vi "Add Small Noise.vi"(11 "channel 1":T2) -> (3 "channel 2":T1)   [LabVIEW 2019]
doc: "Given a value coming in on a channel, disturb that value by a small amount of noise."
uses:
  <extravilib>/ChannelInstances/Stream-i32/)Channel.ctl
  <extravilib>/ChannelInstances/Stream-dbl/)Channel.ctl
  <extravilib>/ChannelInstances/Stream-i32/Read With Abort.vi
  <extravilib>/ChannelInstances/Stream-dbl/Write With Abort.vi
  <extravilib>/ChannelInstances/Stream-i32/EndpointRead.vi
  <extravilib>/ChannelInstances/Stream-dbl/Endpoint.vi
  <extravilib>/ChannelInstances/Stream-i32/)Channel.vi
  <resource>/ChannelSupport/_ChannelSupport/WaitIfNeeded.vi
  <extravilib>/ChannelInstances/Stream-dbl/)Channel.vi
  <extravilib>/ChannelInstances/Stream-i32.lvlib
  <extravilib>/ChannelInstances/Stream-dbl.lvlib
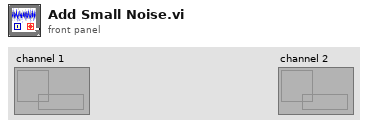
[diagram p1: front panel]
types:
  T1 = typedef "Stream-dbl.lvlib/)Channel.ctl" = refnum<queue>
  T2 = typedef "Stream-i32.lvlib/)Channel.ctl" = refnum<queue>
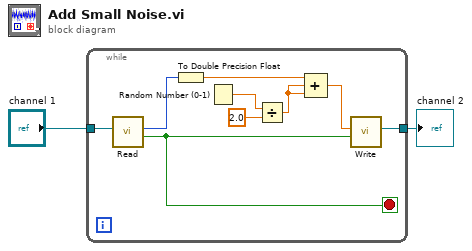
[diagram p0: block diagram]
diagram:
  n1 = while {
    tunnel: [w7] -> w1
    tunnel: "channel 1" -> [w10]
    stop <- w8 stop-if-true
    n2 = call <extravilib>:"Read.vi"("channel"=w10) -> ("last element?"=w8:bool, "element"=w9:i32)  [unwired: 6 in, 3 out]
    n3 = To Double Precision Float(number=w9) -> (double precision float=w3:dbl)
    n4 = Random Number (0-1)() -> (number: 0 to 1=w5:dbl)
    n5 = Divide(x=w5, y=2.0) -> (x/y=w4:dbl)
    n6 = Compound Arithmetic op=ADD(w3, w4, w4) -> (w11:dbl)
    n7 = call <extravilib>:"Write.vi"("last element? (F)"=w8, "element"=w11) -> ("channel"=w7:T1)  [unwired: 7 in, 2 out]
  }
  "channel 2" <- w1
